vi "DriveStraight.vi"(9 "Angle":dbl, 10 "Velocity":dbl) -> ()   [LabVIEW 2016, in "DriveBase.lvclass"]
uses:
  DriveBase.lvclass
  DriveStates.ctl
panel:
  out "error out":errorcluster
  in  "error in (no error)":errorcluster
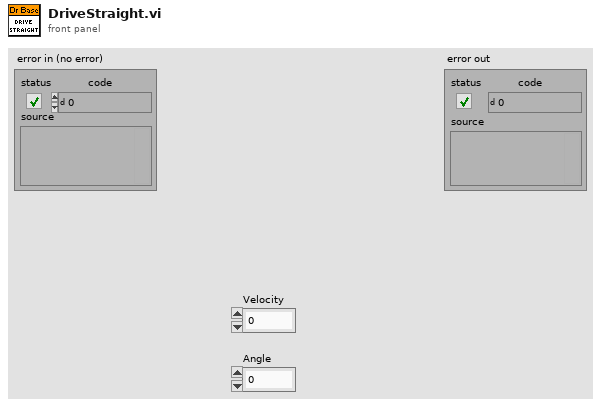
[diagram p1: front panel]
types:
  T1 = typedef "DriveBase.lvclass/DriveStates.ctl" = enum16{"Tank", "Arcade", "DriveStraight"}
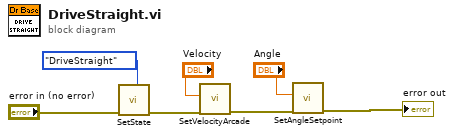
[diagram p0: block diagram]
diagram:
  n1 = call "SetState.vi"("error in (no error)"="error in (no error)", "State"=DriveStates."DriveStraight") -> ("error out"=w3:errorcluster)  [unwired: 9 in]
  n2 = call "SetVelocityArcade.vi"("error in (no error)"=w3, "X Axis"="Velocity") -> ("error out"=w5:errorcluster)  [unwired: 9 in]
  n3 = call "SetAngleSetpoint.vi"("error in (no error)"=w5, "angleSetpointInput"="Angle") -> ("error out"=→"error out":errorcluster)  [unwired: 9 in]
